vi "_TEST Database.vi"(8 "error in (no error)":errorcluster) -> (0 "error out":errorcluster)   [LabVIEW 2011]
panel:
  # "Run Me to Test Database"
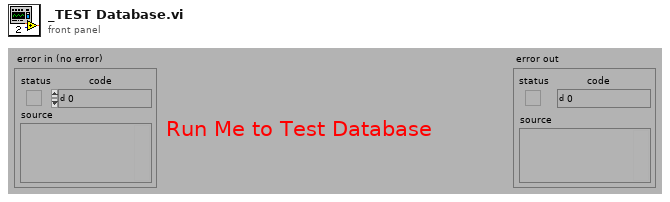
[diagram p1: front panel]
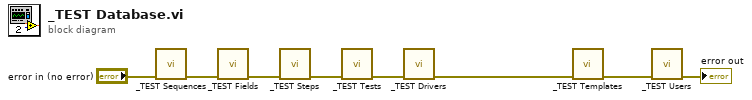
[diagram p0: block diagram]
diagram:
  n1 = call "_TEST Sequences.vi"("error in (no error)"="error in (no error)") -> ("error out"=w8:errorcluster)  [unwired: 6 out]
  n2 = call "_TEST Fields.vi"("error in (no error)"=w8) -> ("error out"=w7:errorcluster)  [unwired: 6 out]
  n3 = call "_TEST Steps.vi"("error in (no error)"=w7) -> ("error out"=w6:errorcluster)  [unwired: 6 out]
  n4 = call "_TEST Tests.vi"("error in (no error)"=w6) -> ("error out"=w5:errorcluster)  [unwired: 6 out]
  n5 = call "_TEST Drivers.vi"("error in (no error)"=w5) -> ("error out"=w1:errorcluster)  [unwired: 6 out]
  n6 = call "_TEST Templates.vi"("error in (no error)"=w1) -> ("error out"=w4:errorcluster)  [unwired: 6 out]
  n7 = call "_TEST Users.vi"("error in (no error)"=w4) -> ("error out"=→"error out":errorcluster)  [unwired: 6 out]
